vi "myRIO_BRIG_FPGA_calc_k2ANDk3.vi"(9 "input_k1[count/ms]":fxp<+,16,16>, 10 "input_Npts":fxp<+,7,7>, 11 "input_freq[kHz]":u8) -> (2 "output_k3":fxp<+,18,4>, 3 "output_k2":u32)   [LabVIEW 2014]
uses:
  <vilib>/rvi/FXPMathLib/FxpDiv/subVIs/nifxpmath_Div_SimConfig.ctl
  <vilib>/rvi/FXPMathLib/FxpDiv/simVIs/DllFxpDivTemp_sub.vi
  <vilib>/rvi/FXPMathLib/FxpMul/XNode/nifxpmath_Multiplier.xnode
  <vilib>/rvi/FXPMathLib/FxpDiv/XNode/nifxpmath_Div.xnode
  <vilib>/rvi/FXPMathLib/sim/FxpSim.dll
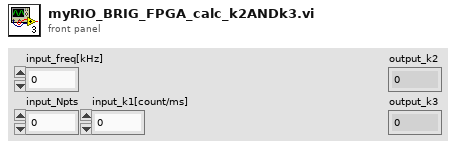
[diagram p1: front panel]
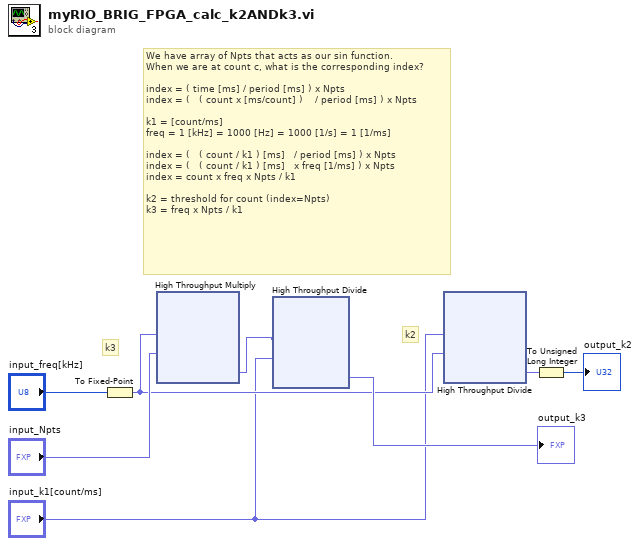
[diagram p0: block diagram]
diagram:
  # "We have array of Npts that acts as our sin function.\nWhen we are at count c, what is the corresponding index?\n\nindex = ( time [ms] / period [ms] ) x Npts\nindex = (   ( count x [ms/count] )    / period [ms] ) x Npts\n\nk1 = [count/ms]\nfreq = 1 [kHz] = 1000 [Hz] = 1000 [1/s] = 1 [1/ms]\n\nindex = (   ( count / k1 ) [ms]   / period [ms] ) x Npts\nindex = (   ( count / k1 ) [ms]   x freq [1/ms] ) x Npts\nindex = count x freq x Npts / k1\n\nk2 = threshold for count (index=Npts)\nk3 = freq x Npts / k1"
  # "k2"
  # "k3"
  n1 = To Fixed-Point(number="input_freq[kHz]") -> (fixed-point=w3:fxp<+,4,4>)  [unwired: 1 in]
  n2 = xnode "High Throughput Multiply"("x"=w3, "y"="input_Npts") -> ("x*y"=w5:fxp<+,11,11>)
  n3 = xnode "High Throughput Divide"("x"=w5, "y"="input_k1[count/ms]") -> ("x/y"=→"output_k3":fxp<+,18,4>)
  n4 = xnode "High Throughput Divide"("x"="input_k1[count/ms]", "y"=w3) -> ("x/y"=w2:fxp<+,16,16>)
  n5 = To Unsigned Long Integer(number=w2) -> (unsigned 32bit integer=→"output_k2":u32)
